vi "Write To File Util.vi"(4 "Maximum File Size (Bytes)":i32=1048576, 5 "Data File Extension":string="dat", 6 "Working Directory":path, 7 "Data File Prefix":string="data", 8 "error in":errorcluster, 9 "Data":dbl[][](array[numeric]) format="%.2f", 10 "Write To File":bool, 11 "File Refnum In":refnum<file>) -> (0 "error out":errorcluster, 2 "Current Data File":path, 3 "File Refnum Out":refnum<file>)   [LabVIEW 2022 SP3]
panel:
  out "File Size (Bytes)":i32
  # "If \"Write To File\" is true, and the refnum points to a closed or otherwise invalid file,\nthen a new file is opened and the data array is written.  When opening, a sequential\nnumber is added to the data file prefix to make unique file names.\n\nIf \"Write To File\" is true, and the refnum points to a valid and open file, the input\ndata array is appended to that file.  Then if the file is bigger than the max size, it\nis closed.\n\nIf \"Write To File\" is false, a close is done on file referenced by the refnum.\n\nThe \"File Refnum\" is created by this VI.  This VI passes the refnum out, and then the\ncalling VI needs to pass the refnum back in so this VI can work with the same file.\nGenerally, that means that the calling VI simply uses a shift register in the loop that\nis calling this VI."
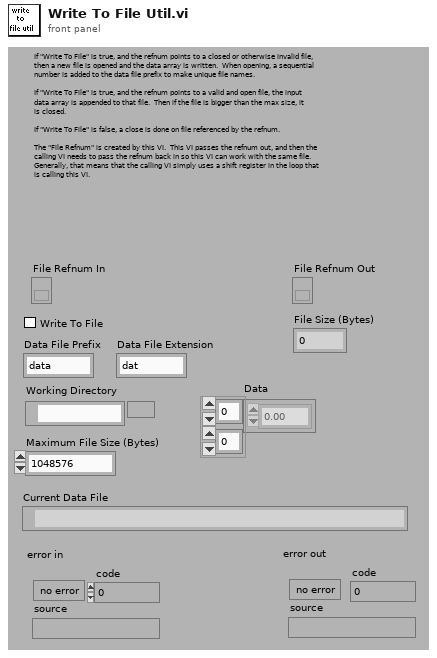
[diagram p1: front panel]
types:
  T1 = enum16{"open", "replace", "create", "open or create", "replace or create", "replace or create with confirmation"}
  T2 = enum16{"deny read/write", "deny write-only", "deny none"}
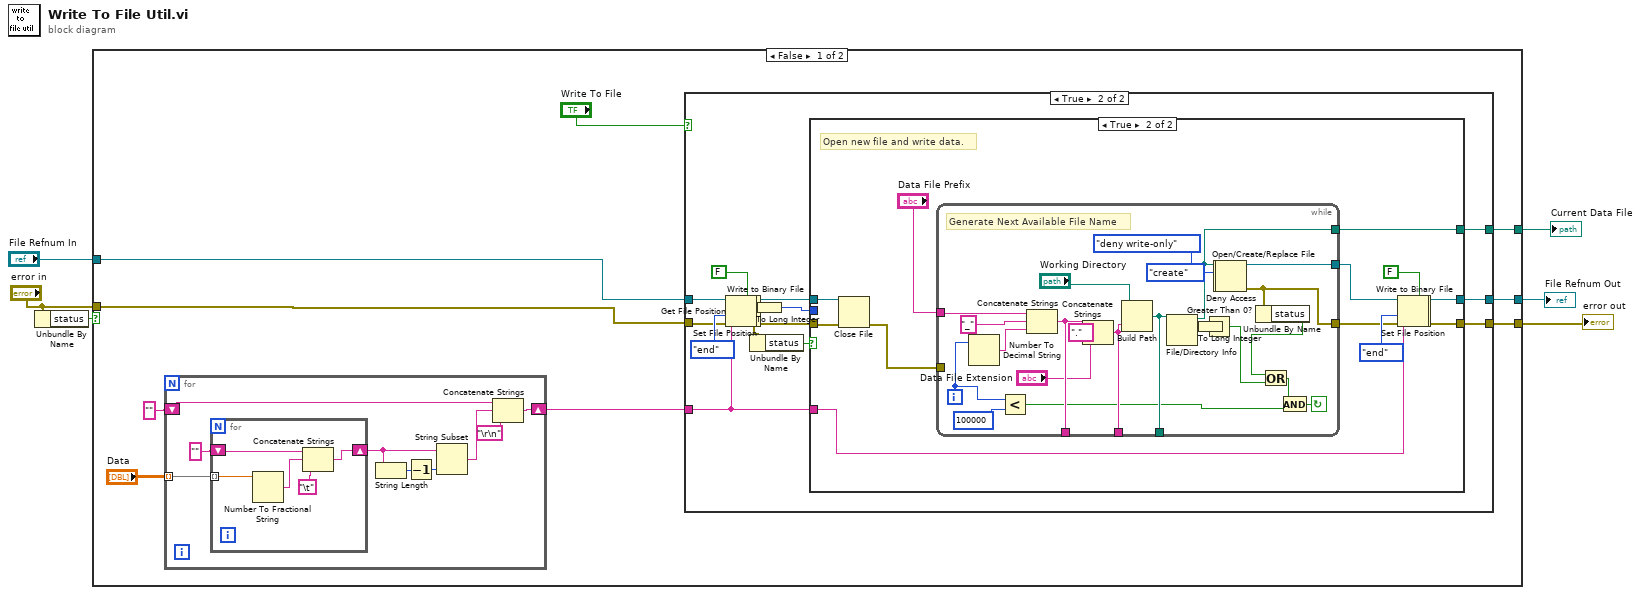
[diagram p0: block diagram]
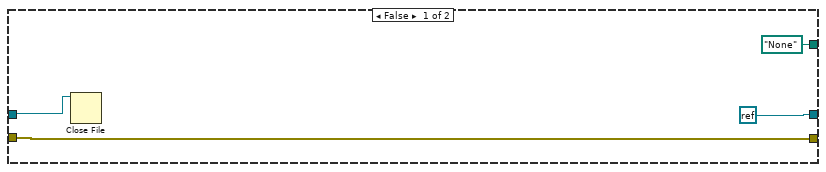
[diagram p2: hidden frame]
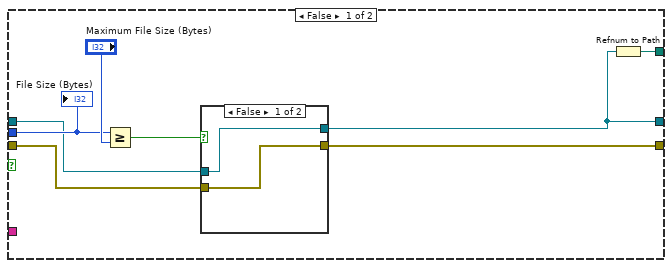
[diagram p3: hidden frame]
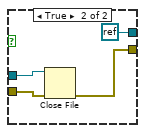
[diagram p4: hidden frame]
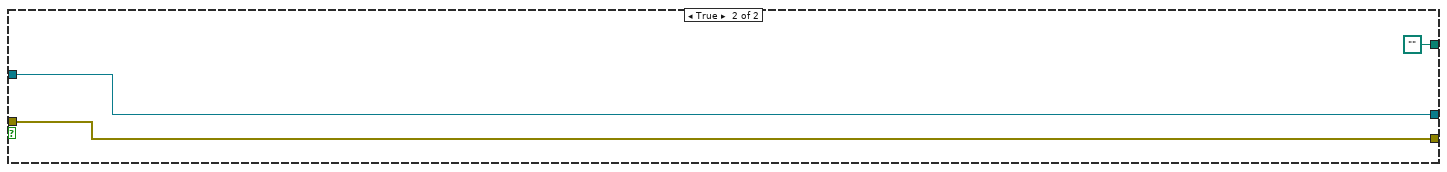
[diagram p5: hidden frame]
diagram:
  n1 = Unbundle By Name("error in") -> ("status"=w2:bool)
  n2 = case shown="False" w2 {
    tunnel: [w15 w105] -> w6
    tunnel: [w14 w104] -> w5
    tunnel: [w9 path "" ("dup path")] -> w4
    tunnel: "File Refnum In" -> [w8 w105]
    tunnel: "error in" -> [w7 w104]
    frame False {
      n3 = for {
        tunnel: "Data" -> [w24] mode=indexing
        shift-right: [w20] -> w10
        shift-left: "" -> [w19]
        n4 = for {
          shift-right: [w26] -> w21
          shift-left: "" -> [w27]
          tunnel: w24 -> [w29] mode=indexing
          n5 = Number To Fractional String(number=w29) -> (F-format string=w28:string)  [unwired: 3 in]
          n6 = Concatenate Strings(w27, w28, "\t") -> (w26:string)
        }
        n7 = String Length(string=w21) -> (length=w22:i32)
        n8 = Decrement(x=w22) -> (x-1=w23:i32)
        n9 = String Subset(string=w21, length (rest)=w23) -> (substring=w18:string)  [unwired: 1 in]
        n10 = Concatenate Strings(w19, w18, "\r\n") -> (w20:string)
      }
      n11 = case shown="True" "Write To File" {
        tunnel: [refnum<k0> refnum w47] -> w15
        tunnel: [w30 w46] -> w14
        tunnel: w8 -> [w33 w45]
        tunnel: w7 -> [w30 w44]
        tunnel: w10 -> [_ w43]
        tunnel: [path "None" ("dup path") w42] -> w9
        frame False {
          n12 = Close File(refnum=w33) -> ()  [unwired: 1 in, 2 out]
        }
        frame True {
          n13 = Set File Position(refnum=w45, from (0:start)=enum16{"start", "end", "current"}."end" ("pos mode (0:2)"), error in=w44) -> (refnum out=w39:refnum<file>, error out=w38:errorcluster)  [unwired: 1 in]
          n14 = Write to Binary File(file (use dialog)=w39, data=w43, error in=w38, 5:FALSE ("prepend array or string size? (T)")) -> (refnum out=w37:refnum<file>, error out=w36:errorcluster)  [unwired: 2 in, 1 out]
          n15 = Get File Position(4:w36, 7:w37) -> (0:w41:errorcluster, 2:w35:i64, 3:w48:refnum<file>)
          n16 = Unbundle By Name(w41) -> ("status"=w40:bool)
          n17 = To Long Integer(number=w35) -> (32bit integer=w49:i32)
          n18 = case shown="True" w40 {
            tunnel: w49 -> [w57 _]
            tunnel: w48 -> [w55 w77]
            tunnel: [w56 w74] -> w46
            tunnel: [w52 w71] -> w47
            tunnel: w43 -> [_ w70]
            tunnel: [w53 w69] -> w42
            tunnel: w41 -> [w51 w68]
            frame False {
              n19 = Greater Or Equal?(x=w57, y="Maximum File Size (Bytes)") -> (x >= y?=w54:bool)
              n20 = case shown="False" w54 {
                tunnel: [w60 w64] -> w56
                tunnel: w51 -> [w60 w63]
                tunnel: w55 -> [w59 w62]
                tunnel: [w59 refnum<k0> refnum] -> w52
                frame False {
                }
                frame True {
                  n21 = Close File(refnum=w62, error in=w63) -> (error out=w64:errorcluster)  [unwired: 1 out]
                }
              }
              n22 = Refnum to Path(1:w52) -> (0:w53:path)
              "File Size (Bytes)" <- w57
            }
            frame True {
              # "Open new file and write data."
              n23 = Close File(refnum=w77, error in=w68) -> (error out=w76:errorcluster)  [unwired: 1 out]
              n24 = while {
                tunnel: [w83] -> w69
                tunnel: [w84] -> w73
                tunnel: w76 -> [_]
                tunnel: [w92] -> w72
                tunnel: [w98] -> _
                tunnel: [w94] -> _
                tunnel: [w99] -> _
                tunnel: "Data File Prefix" -> [w101]
                i -> [w88]
                stop <- w85 continue-if-true
                # "Generate Next Available File Name"
                n25 = Number To Decimal String(number=w88) -> (decimal integer string=w103:string)  [unwired: 1 in]
                n26 = Less?(x=w88, y=100000) -> (x < y?=w86:bool)
                n27 = Concatenate Strings(w101, "_" ("Substring"), w103) -> (w98:string)
                n28 = Concatenate Strings(w98, "." ("Substring"), "Data File Extension") -> (w99:string)
                n29 = Build Path(base path="Working Directory", name or relative path=w99) -> (appended path=w94:path)
                n30 = File/Directory Info(path=w94) -> (path out=w83:path, size=w82:i64)  [unwired: 1 in, 5 out]
                n31 = To Long Integer(number=w82) -> (32bit integer=w102:i32)
                n32 = Greater Than 0?(x=w102) -> (x > 0?=w97:bool)
                n33 = Open/Create/Replace File(file path (use dialog)=w83, operation (0:open)=T1."create") -> (refnum out=w80:refnum<file>, error out=w81:errorcluster)  [unwired: 4 in, 1 out]
                n34 = Deny Access(4:w81, 6:T2."deny write-only" ("deny mode (2)"), 7:w80) -> (0:w84:errorcluster, 3:w92:refnum<file>)
                n35 = Unbundle By Name(w84) -> ("status"=w96:bool)
                n36 = Or(x=w96, y=w97) -> (x .or. y?=w89:bool)
                n37 = And(x=w89, y=w86) -> (x .and. y?=w85:bool)
              }
              n38 = Set File Position(refnum=w72, from (0:start)=enum16{"start", "end", "current"}."end" ("pos mode (0:2)"), error in=w73) -> (refnum out=w67:refnum<file>, error out=w66:errorcluster)  [unwired: 1 in]
              n39 = Write to Binary File(file (use dialog)=w67, data=w70, error in=w66, 5:FALSE ("prepend array or string size? (T)")) -> (refnum out=w71:refnum<file>, error out=w74:errorcluster)  [unwired: 2 in, 1 out]
            }
          }
        }
      }
    }
    frame True {
    }
  }
  "error out" <- w5
  "File Refnum Out" <- w6
  "Current Data File" <- w4
